vi "test - docs pure English.vi"(8 "error in (no error)":errorcluster, 11 "TestCase in":refnum<class "testcase-documentation.lvclass">) -> (0 "error out":errorcluster, 3 "TestCase out":refnum<class "testcase-documentation.lvclass">)   [LabVIEW 2017, in "testcase-documentation.lvclass"]
uses:
  testcase-documentation.lvclass
  <vilib>/addons/_JKI Toolkits/VI Tester/TestCase.llb/TestCase.lvclass
  src/user.lib/_NEVSTOP/Communicable State Machine(CSM)/_csmDoc/csmdoc.lvlib
  src/user.lib/_NEVSTOP/Communicable State Machine(CSM)/_Shared/CSM Shared.lvlib
  src/user.lib/_NEVSTOP/Communicable State Machine(CSM)/Communicable State Machine.lvlib
  C:/Program Files (x86)/National Instruments/LabVIEW 2017/vi.lib/addons/_JKI Toolkits/VI Tester/TestCase.llb/TestCase.lvclass
panel:
  out "Array 3":string[](array[string])
  out "Array 2":u8[](array[numeric])
  out "Array":string[](array[string])
  out "size(s)":i32
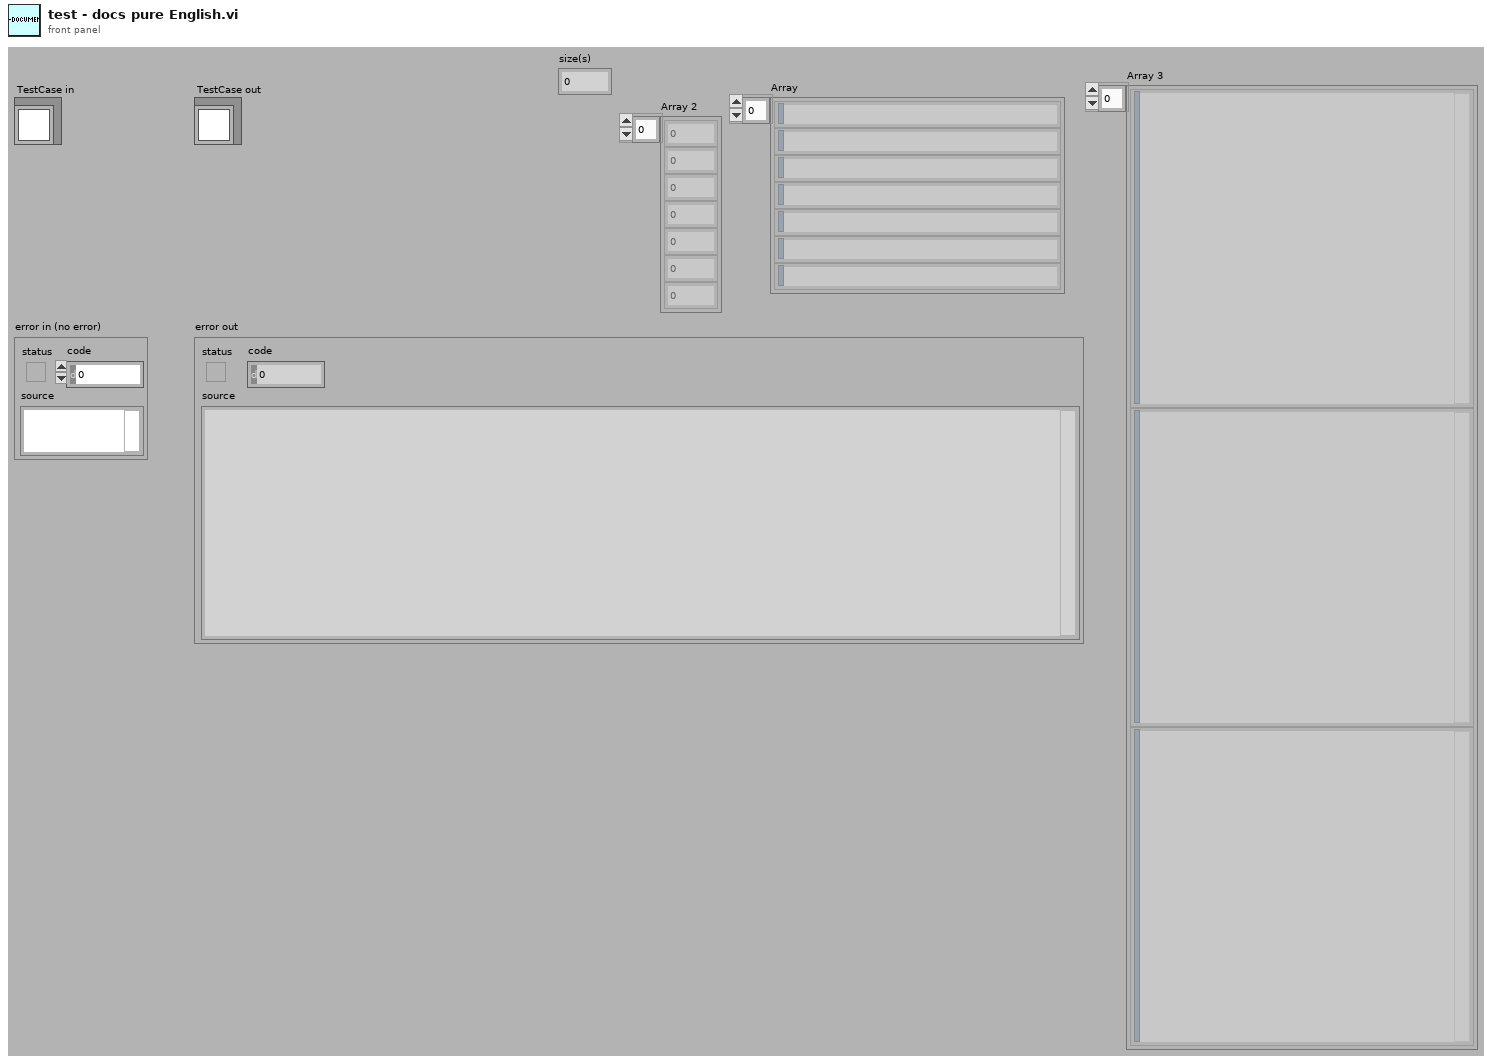
[diagram p1: front panel]
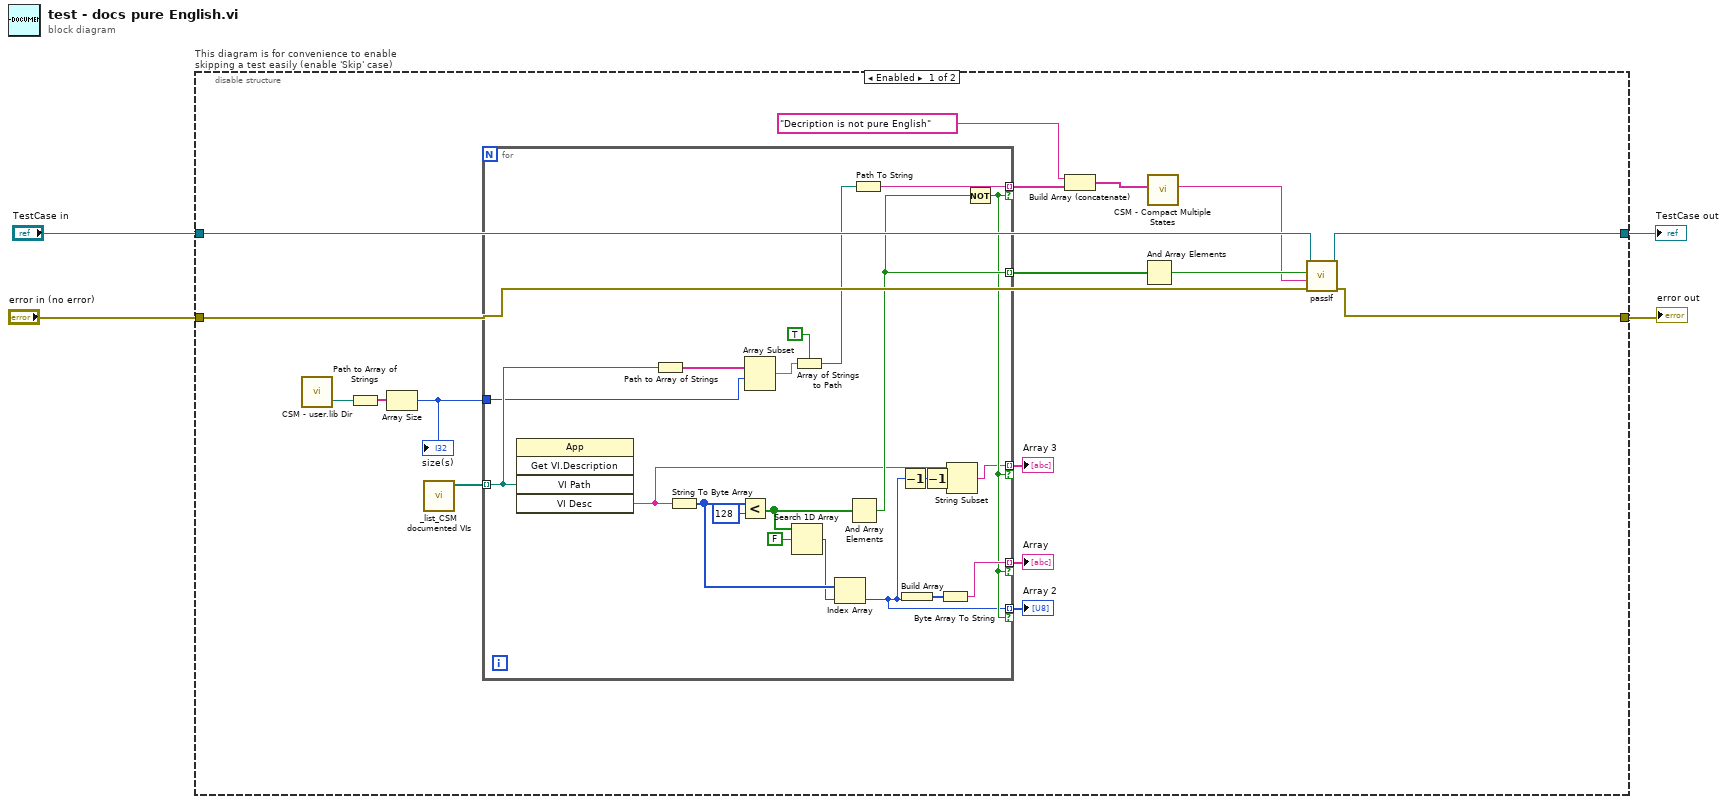
[diagram p0: block diagram]
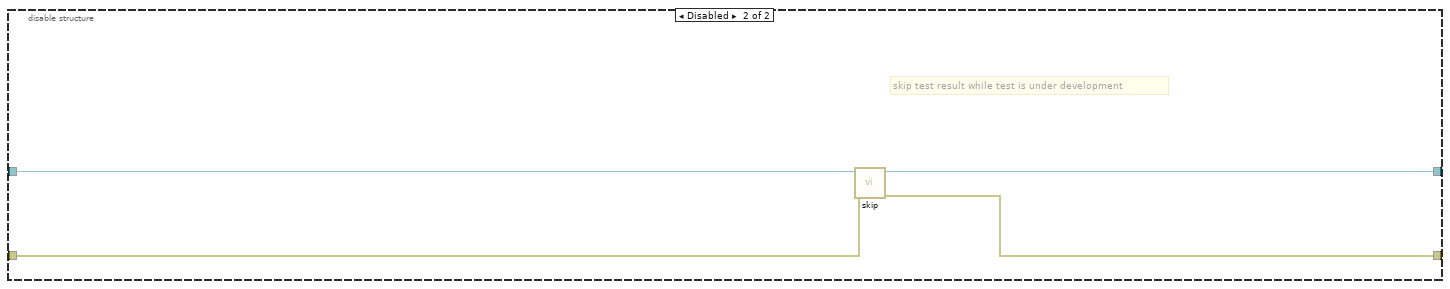
[diagram p2: hidden frame]
diagram:
  n1 = disable-structure "This diagram is for convenience to enable skipping a test easily (enable 'Skip' case)" shown="Enabled" {
    disable-tunnel: "TestCase in" -> [w21 w46]
    disable-tunnel: [w20 w44] -> w1
    disable-tunnel: [w19 w45] -> w3
    disable-tunnel: "error in (no error)" -> [w18 w43]
    frame Enabled {
      n2 = call "CSM - user.lib Dir.vi"() -> ("<LabVIEW>"=w15:path)  [unwired: 2 in, 1 out]
      n3 = Path to Array of Strings(0:w15) -> (2:w16:string[])  [unwired: 1 out]
      n4 = Array Size(array=w16) -> (size(s)=w14:i32)
      "size(s)" <- w14
      n5 = call "_list_CSM documented VIs.vi"() -> ("Array"=w17:path[])  [unwired: 11 in]
      n6 = for {
        tunnel: w17 -> [w42] mode=indexing
        tunnel: w14 -> [w41]
        tunnel: [w34] -> w13 mode=indexing
        tunnel: [w39] -> w12 mode=indexing if=w27
        tunnel: [w28] -> w7 mode=indexing if=w27
        tunnel: [w24] -> w6 mode=indexing if=w27
        tunnel: [w26] -> w5 mode=indexing if=w27
        n7 = invoke class="App" method="Get VI.Description"("VI Path"=w42) -> ("VI Desc"=w25:string)  [unwired: 4 in, 4 out]
        n8 = Path to Array of Strings(0:w42) -> (2:w36:string[])  [unwired: 1 out]
        n9 = String To Byte Array(string=w25) -> (unsigned byte array=w31:u8[])
        n10 = Less?(x=w31, y=u8 128) -> (x < y?=w33:bool[])
        n11 = Array Subset(array=w36, index=w41) -> (w38:string[])  [unwired: 1 in]
        n12 = Search 1D Array(1D array=w33, element=FALSE) -> (index of element=w30:i32)  [unwired: 1 in]
        n13 = Array of Strings to Path(0:w38, 1:TRUE ("relative")) -> (2:w35:path)
        n14 = Index Array(array=w31, index=w30) -> (element=w24:u8)
        n15 = And Array Elements(Boolean array=w33) -> (logical AND=w34:bool)
        n16 = Path To String(path=w35) -> (string=w39:string)
        n17 = Decrement(x=w24) -> (x-1=w23:u8)
        n18 = Build Array(w24) -> (w29:u8[])
        n19 = Decrement(x=w23) -> (x-1=w22:u8)
        n20 = Byte Array To String(unsigned byte array=w29) -> (string=w28:string)
        n21 = String Subset(string=w25, offset (0)=w22) -> (substring=w26:string)  [unwired: 1 in]
        n22 = Not(x=w34) -> (.not. x?=w27:bool)
      }
      "Array" <- w7
      "Array 2" <- w6
      "Array 3" <- w5
      n23 = Build Array (concatenate)("Decription is not pure English" ("message (\"\")"), w12) -> (w10:string[])
      n24 = And Array Elements(Boolean array=w13) -> (logical AND=w11:bool)
      n25 = call "CSM - Compact Multiple States.vi"("Multiple States"=w10) -> ("States"=w8:string)  [unwired: 9 in]
      n26 = call-dynamic "passIf.vi"("error in (no error)"=w18, "message (\"\")"=w8, "pass"=w11, "TestCase in"=w21) -> ("error out"=w19:errorcluster, "TestCase out"=w20:refnum<class "testcase-documentation.lvclass">)  [unwired: 6 in]
    }
    frame Disabled {
      # "skip test result while test is under development"
      n27 = call <vilib>:"skip.vi"("error in (no error)"=w43, "TestCase in"=w46) -> ("error out"=w45:errorcluster, "TestCase out"=w44:refnum<class "testcase-documentation.lvclass">)  [unwired: 8 in]
    }
  }
  "error out" <- w3
  "TestCase out" <- w1
